vi "ReadJson.vi"(8 "error in (no error)":errorcluster, 11 "json object":string) -> (0 "error out":errorcluster, 3 "json string":string)   [LabVIEW 2017, in "GlobalConfiguration.lvlib"]
uses:
  <vilib>/addons/InsightCM/Utilities/GlobalConfiguration/GlobalConfiguration.lvlib
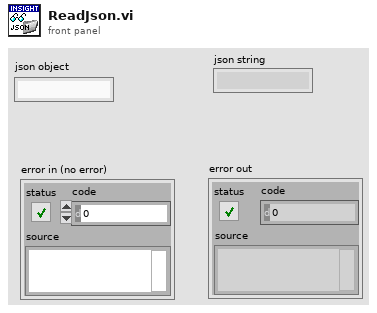
[diagram p1: front panel]
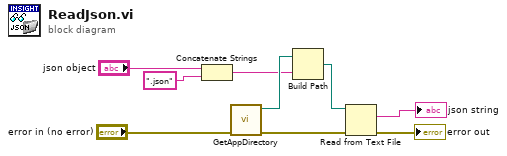
[diagram p0: block diagram]
diagram:
  n1 = Concatenate Strings("json object", ".json" ("string")) -> (w2:string)
  n2 = call <vilib>:"GetAppDirectory.vi"("error in (no error)"="error in (no error)") -> ("error out"=w5:errorcluster, "application directory"=w6:path)  [unwired: 9 in]
  n3 = Build Path(base path=w6, name or relative path=w2) -> (appended path=w9:path)
  n4 = Read from Text File(file (use dialog)=w9, error in=w5) -> (text=→"json string":string, error out=→"error out":errorcluster)  [unwired: 2 in, 2 out]
